vi "Count Particles.vi"(8 "error in":errorcluster, 10 "Channel Index":u16, 11 "Live Frame":u16[][][](array[numeric])) -> (0 "error out":errorcluster, 2 "Numeric":dbl, 3 "String":string)   [LabVIEW 2023, in "Viewer.lvlib"]
uses:
  Viewer.lvlib
panel:
  out "Elapsed (s)":dbl
  in  "Use DLL?":bool
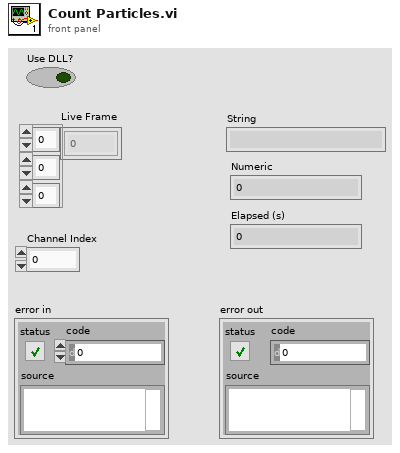
[diagram p1: front panel]
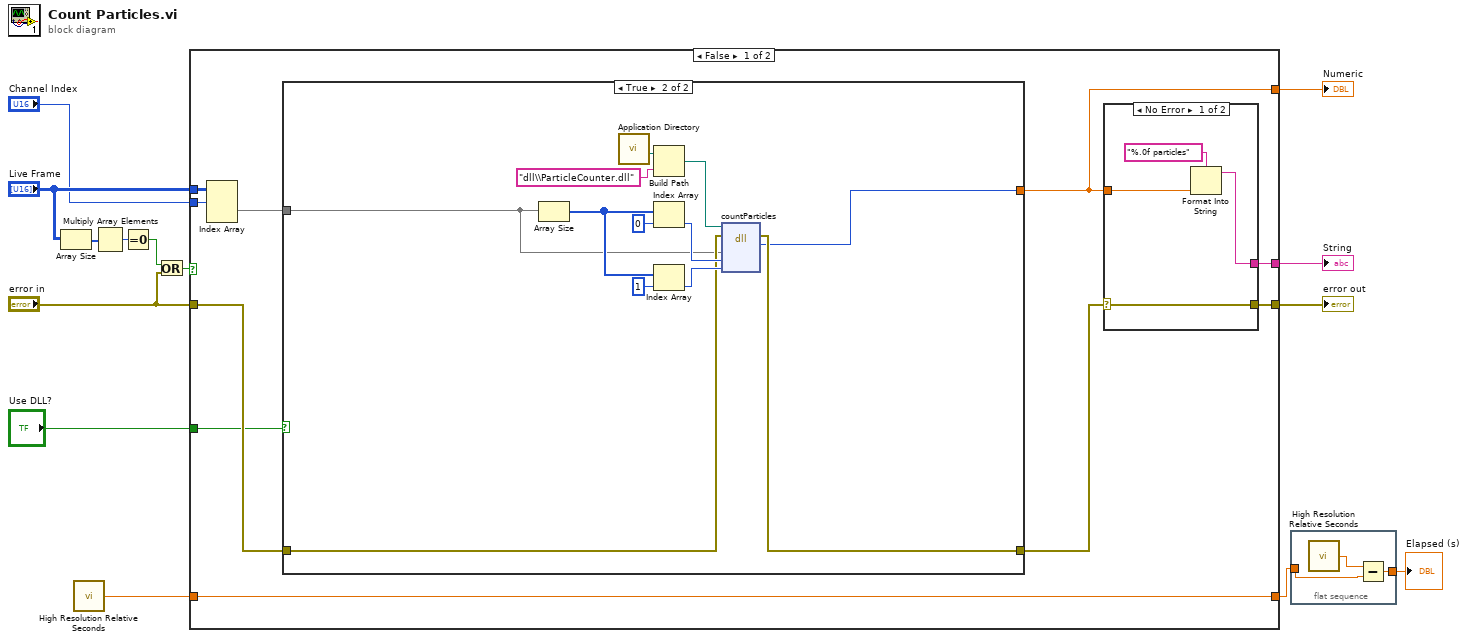
[diagram p0: block diagram]
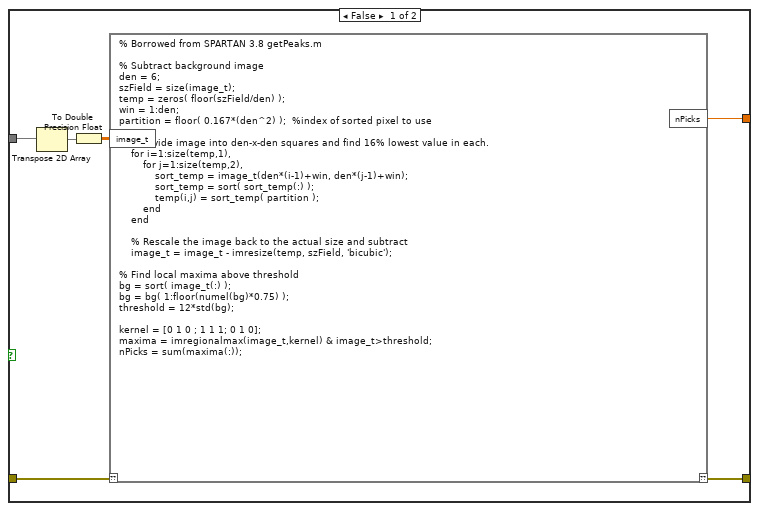
[diagram p2: hidden frame]
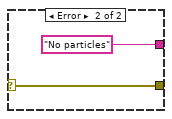
[diagram p3: hidden frame]
diagram:
  n1 = Array Size(array="Live Frame") -> (size(s)=w9:i32[])
  n2 = call <vilib>:"High Resolution Relative Seconds.vi"() -> ("relative seconds"=w2:dbl)
  n3 = Multiply Array Elements(1:w9) -> (0:w8:i32)
  n4 = Equal To 0?(x=w8) -> (x = 0?=w6:bool)
  n5 = Or(x=w6, y="error in") -> (x .or. y?=w11:bool)
  n6 = case shown="False" w11 {
    tunnel: "Live Frame" -> [w24 _]
    tunnel: [w23 _] -> w13
    tunnel: [w17 w50] -> w14
    tunnel: [w22 _] -> w12
    tunnel: "error in" -> [w21 w50]
    tunnel: "Channel Index" -> [w19 _]
    tunnel: "Use DLL?" -> [w16 _]
    tunnel: w2 -> [w15 w49]
    tunnel: [w15 w49] -> w1
    frame False {
      n7 = Index Array(array=w24, index (dim 0)=w19) -> (element=w20:u16[][])  [unwired: 2 in]
      n8 = case shown="True" w16 {
        tunnel: [w29 w34] -> w22
        tunnel: w21 -> [w28 w37]
        tunnel: w20 -> [w27 w35]
        tunnel: [w25 w36] -> w18
        frame False {
          n9 = Transpose 2D Array(2D array=w27) -> (transposed array=w26:u16[][])
          n10 = To Double Precision Float(number=w26) -> (double precision float=w30:dbl[][])
          n11 = script code="% Borrowed from SPARTAN 3.8 getPeaks.m\n\n% Subtract background image\nden = 6;\nszField = size(image_t);\ntemp = zeros( floor(szField/den) );\nwin = 1:den;\npartition = floor( 0.167*(den^2) );  %index of sorted pixel to use\n\n    % Divide image into den-x-den squares and find 16% lowest value in each.\n    for i=1:size(temp,1),\n        for j=1:size(temp,2),\n            sort_temp = image_t(den*(i-1)+win, den*(j-1)+win);\n            sort_temp = sort( sort_temp(:) );\n            temp(i,j) = sort_temp( partition );\n        end\n    end\n    \n    % Rescale the image back to the actual size and subtract\n    image_t = image_t - imresize(temp, szField, 'bicubic');\n\n% Find local maxima above threshold\nbg = sort( image_t(:) );\nbg = bg( 1:floor(numel(bg)*0.75) );\nthreshold = 12*std(bg);\n\nkernel = [0 1 0 ; 1 1 1; 0 1 0];\nmaxima = imregionalmax(image_t,kernel) & image_t>threshold;\nnPicks = sum(maxima(:));"("??"=w28, "image_t"=w30) -> ("??"=w25:errorcluster, "nPicks"=w29:dbl)
        }
        frame True {
          n12 = Array Size(array=w35) -> (size(s)=w39:i32[])
          n13 = call <vilib>:"Application Directory.vi"() -> ("Application Directory"=w33:path)
          n14 = Build Path(base path=w33, name or relative path="dll\\ParticleCounter.dll") -> (appended path=w31:path)
          n15 = Index Array(array=w39, index=0) -> (element=w41:i32)
          n16 = Index Array(array=w39, index=1) -> (element=w38:i32)
          n17 = dll-call lib="?" fn="countParticles"(path in=w31, error in=w37, "data"=w35, "rows"=w41, "cols"=w38) -> (error out=w36:errorcluster, "return type"=w34:u32)  [unwired: 4 in, 1 out]
        }
      }
      n18 = case shown="No Error" w18 {
        selector: w18 -> [w43 w47]
        tunnel: [w45 "No particles"] -> w23
        tunnel: w22 -> [w44 _]
        tunnel: [w43 w47] -> w17
        frame No Error {
          n19 = Format Into String(format string="%.0f particles", w44) -> (resulting string=w45:string)  [unwired: 2 in, 1 out]
        }
        frame Error {
        }
      }
    }
    frame True {
    }
  }
  "error out" <- w14
  "String" <- w13
  "Numeric" <- w12
  n20 = flat-sequence {
    tunnel: w1 -> [w52]
    tunnel: [w51] -> w3
    frame #0 {
      n21 = call <vilib>:"High Resolution Relative Seconds.vi"() -> ("relative seconds"=w53:dbl)
      n22 = Subtract(x=w53, y=w52) -> (x-y=w51:dbl)
    }
  }
  "Elapsed (s)" <- w3
